vi "WaitPassRole.vi"(7 "first call":bool, 9 "Game in":refnum<class "Game.lvclass">, 10 "Tactic index in":i32, 11 "WaitPassRole":refnum<class "WaitPassRole.lvclass">) -> (0 "tactic index":i32, 1 "Game out":refnum<class "Game.lvclass">, 2 "Robot out":refnum<class "Robot.lvclass">, 3 "WaitPassRole out":refnum<class "WaitPassRole.lvclass">)   [LabVIEW 2024, in "WaitPassRole.lvclass"]
uses:
  WaitPassRole.lvclass
  Robot_class/Robot.lvclass
  Game_class/Game.lvclass
  C:/Users/moise/Documents/GitHub/SSL_AI/Role_class/Role.lvclass
  Role_class/Role.lvclass/Role.ctl
  Utilities_class/Utilities.lvclass
  WaitPassRole.lvclass/WaitPassRole.ctl
  Tacticbook_class/Tacticbook.lvclass/Tacticbook.ctl
  Tacticbook_class/Read WaitPassTactic.vi
  Tacticbook_class/Write WaitPassTactic.vi
  Role_class/Read Tacticbook.vi
  Read Number of Tatics.vi
  Role_class/Write Tacticbook.vi
  Role_class/Write tactic_index.vi
  Role_class/Read RobotRef.vi
  Tacticbook_class/Tacticbook.lvclass
  WaitPassTactic_class/WaitPassTactic.lvclass
panel:
  out "error out":errorcluster
  in  "error in (no error)":errorcluster
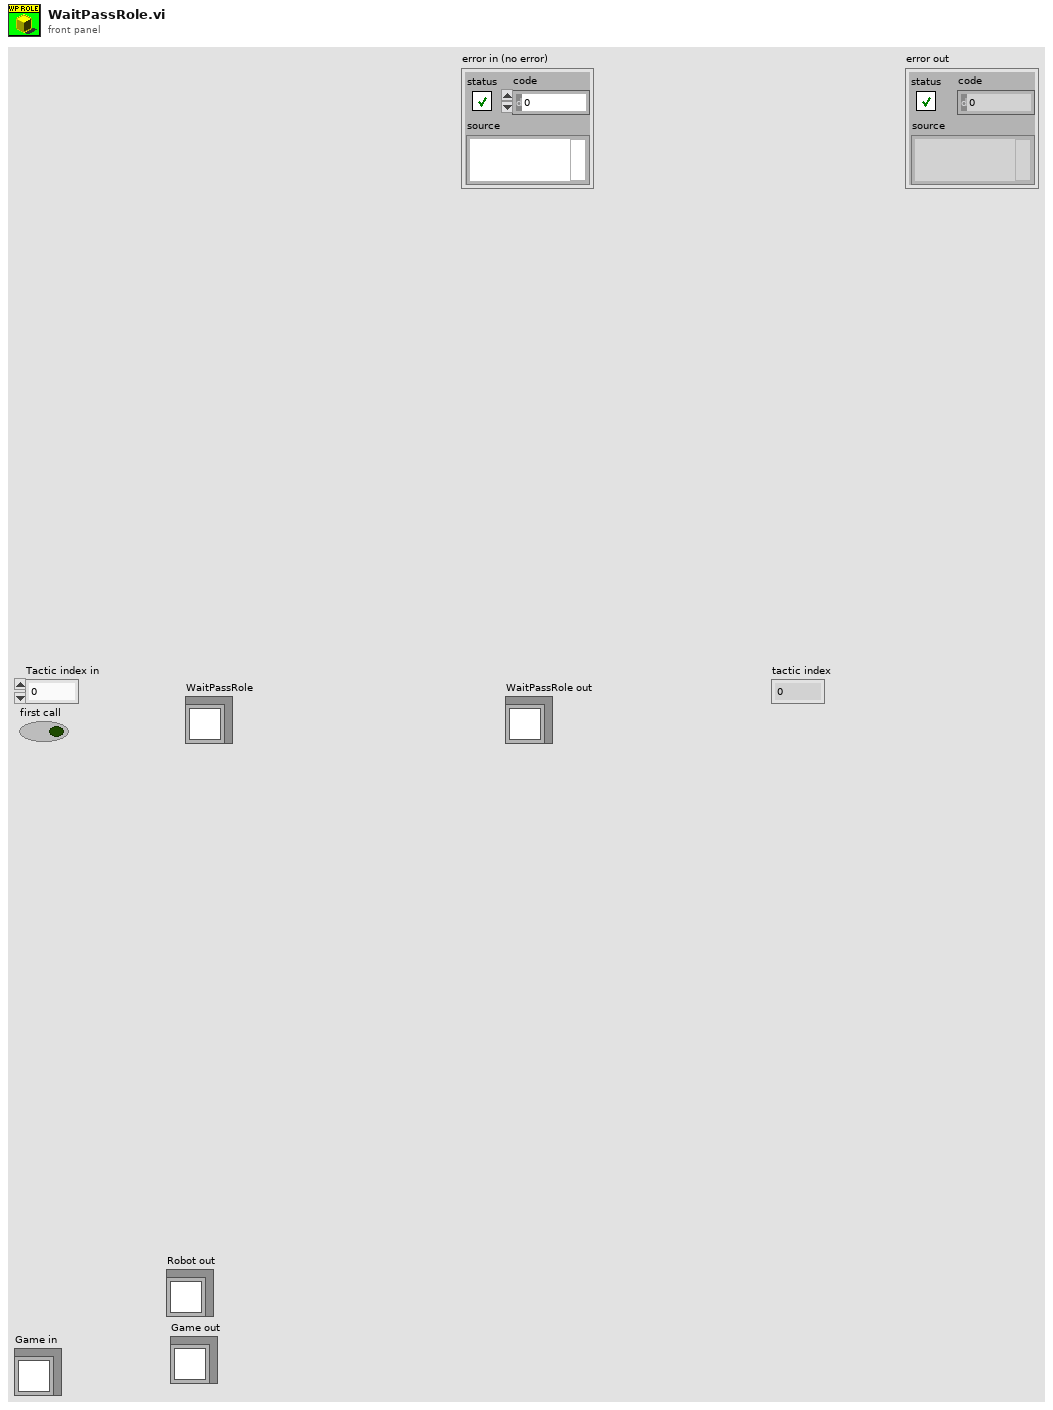
[diagram p1: front panel]
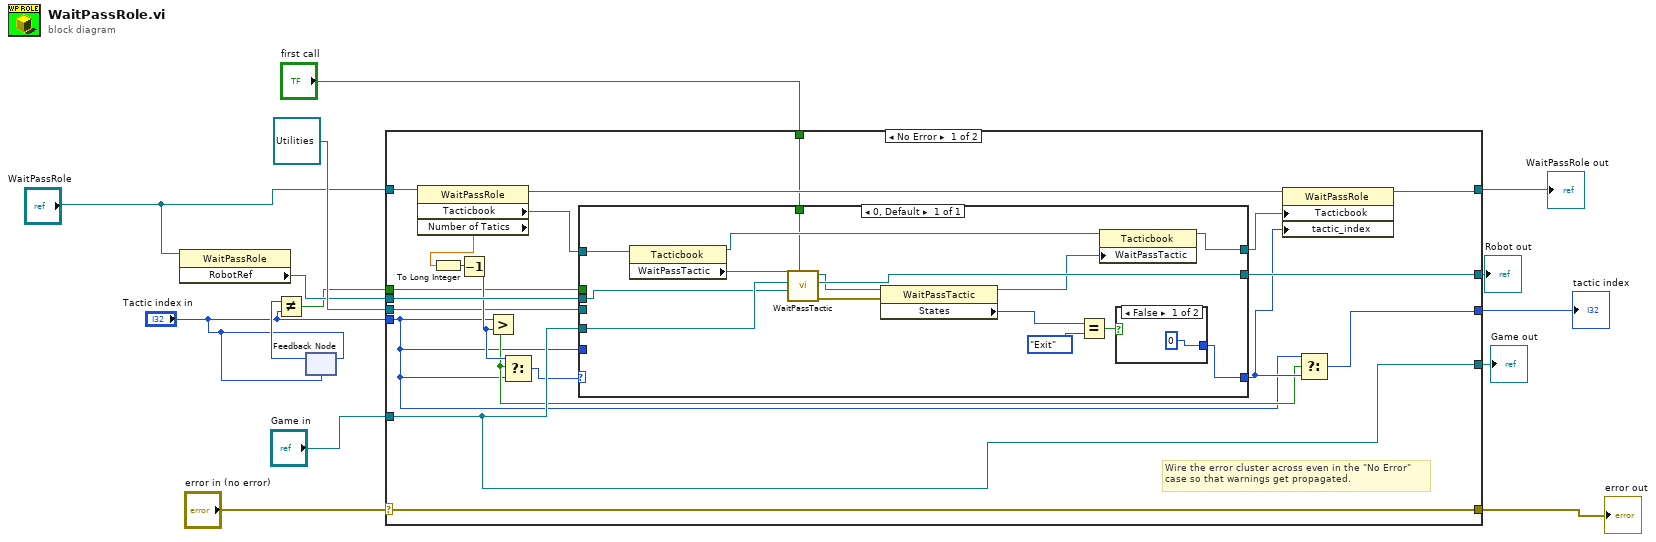
[diagram p0: block diagram]
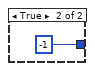
[diagram p2: hidden frame]
diagram:
  n1 = property class="WaitPassRole"(reference="WaitPassRole") -> ("RobotRef"=w7:refnum<class "Robot.lvclass">)  [unwired: 1 in, 2 out]
  n2 = feedback #1("Tactic index in") -> (w5:i32)
  n3 = Not Equal?(x=w5, y="Tactic index in") -> (x != y?=w3:bool)
  n4 = feedback-in #1("Tactic index in") -> ()
  n5 = case shown="No Error" "error in (no error)" {
    selector: "error in (no error)" -> [w34 w55]
    tunnel: [w34 w55] -> w10
    tunnel: [w32 w54] -> w1
    tunnel: "WaitPassRole" -> [w33 w54]
    tunnel: w7 -> [w29 w53]
    tunnel: [w28 w53] -> w14
    tunnel: [w26 w52] -> w13
    tunnel: "Game in" -> [w26 w52]
    tunnel: [w21 _] -> w9
    tunnel: "Tactic index in" -> [w20 _]
    tunnel: refnum<class "Utilities.lvclass"> refnum ("Utilities in") -> [w19 _]
    tunnel: "first call" -> [w18 _]
    tunnel: w3 -> [w15 _]
    frame No Error {
      # "Wire the error cluster across even in the \"No Error\"\ncase so that warnings get propagated."
      n6 = property class="WaitPassRole"(reference=w33) -> (reference out=w31:refnum<class "WaitPassRole.lvclass">, "Tacticbook"=w30:refnum<class "Tacticbook.lvclass">, "Number of Tatics"=w16:dbl)  [unwired: 1 in, 1 out]
      n7 = To Long Integer(number=w16) -> (32bit integer=w17:i32)
      n8 = Decrement(x=w17) -> (x-1=w25:i32)
      n9 = Greater?(x=w20, y=w25) -> (0:w22:bool)
      n10 = Select(t=w25, s=w22, f=w20) -> (s? t:f=w24:i32)
      n11 = case shown="0, Default" w24 {
        tunnel: [w37] -> w23
        tunnel: w30 -> [w49]
        tunnel: w29 -> [w40]
        tunnel: [w48] -> w28
        tunnel: [w44] -> w27
        tunnel: w26 -> [w41]
        tunnel: w20 -> [_]
        tunnel: w19 -> [_]
        tunnel: w18 -> [w36]
        tunnel: w15 -> [_]
        frame 0, Default {
          n12 = property class="Tacticbook"(reference=w49) -> (reference out=w46:refnum<class "Tacticbook.lvclass">, "WaitPassTactic"=w43:refnum<class "WaitPassTactic.lvclass">)  [unwired: 1 in, 1 out]
          n13 = call-dynamic "WaitPassTactic.vi"("first call"=w36, "Robot"=w40, "Game in"=w41, "WaitPassTactic in"=w43) -> ("error out"=w47:errorcluster, "Robot out"=w48:refnum<class "Robot.lvclass">, "WaitPassTactic out"=w42:refnum<class "WaitPassTactic.lvclass">)  [unwired: 5 in]
          n14 = property class="WaitPassTactic"(reference=w42, error in=w47) -> (reference out=w45:refnum<class "WaitPassTactic.lvclass">, "States"=w38:enum16{"State 0", "State 1", "State 2", "Exit"})  [unwired: 1 out]
          n15 = Equal?(x=w38, y=enum16{"State 0", "State 1", "State 2", "Exit"}."Exit") -> (x = y?=w39:bool)
          n16 = property class="Tacticbook"(reference=w46, "WaitPassTactic"=w45) -> (reference out=w44:refnum<class "Tacticbook.lvclass">)  [unwired: 1 in, 1 out]
          n17 = case shown="False" w39 {
            tunnel: [0 -1] -> w37
            frame False {
            }
            frame True {
            }
          }
        }
      }
      n18 = property class="WaitPassRole"(reference=w31, "Tacticbook"=w27, "tactic_index"=w23) -> (reference out=w32:refnum<class "WaitPassRole.lvclass">)  [unwired: 1 in, 1 out]
      n19 = Select(t=w20, s=w22, f=w23) -> (s? t:f=w21:i32)
    }
    frame Error {
    }
  }
  "error out" <- w10
  "Robot out" <- w14
  "Game out" <- w13
  "tactic index" <- w9
  "WaitPassRole out" <- w1
